vi "Sleep TC HL.vi"(8 "error in":errorcluster, 11 "Module ID":i32=-1) -> (0 "error out":errorcluster)   [LabVIEW 2020, in "NI DAQ.lvlib"]
doc: "Request to set the timeout of the TC HL to infinite.\n\n_____\nCreated using DQMH Framework: Event Scripter 7.1.1.1528."
uses:
  NI DAQ.lvlib
  Sleep TC HL Argument--cluster.ctl
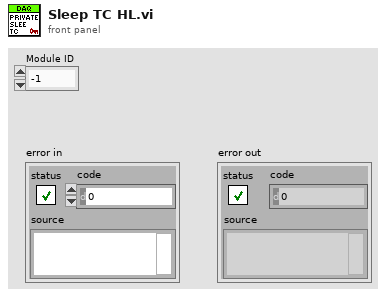
[diagram p1: front panel]
types:
  T1 = typedef "NI DAQ.lvlib/Sleep TC HL Argument--cluster.ctl" = cluster{"Module ID":i32, "Boolean":bool}
  T2 = typedef "NI DAQ.lvlib/Request Events--cluster.ctl" = cluster{"Stop Module":refnum<user-event>, "Show Panel":refnum<user-event>, "Hide Panel":refnum<user-event>, "Show Diagram":refnum<user-event>, "Get Module Execution Status":refnum<user-event>, "Set device name":refnum<user-event>, "Get channel list":refnum<user-event>, "Start task":refnum<user-event>, "Stop task":refnum<user-event>, "Write DO":refnum<user-event>, "Create DI channel":refnum<user-event>, "Read DI":refnum<user-event>, "Get task ref":refnum<user-event>, "Wake up HL":refnum<user-event>, "Sleep HL":refnum<user-event>, "Create AI channel":refnum<user-event>, "Read AI":refnum<user-event>, "Create AO channel":refnum<user-event>, "Write AO":refnum<user-event>, "Validate connection":refnum<user-event>, "Start continous acquisition":refnum<user-event>, "Stop continuous acquisition":refnum<user-event>, "Create DO channel":refnum<user-event>, "Create CI channel":refnum<user-event>, "Read CI":refnum<user-event>, "Get device model":refnum<user-event>, "Get device name":refnum<user-event>, "Create TC channel":refnum<user-event>, "Read TC":refnum<user-event>, "Start Continuous DI":refnum<user-event>, "Local Instance":T3, "Stop continuous DI":refnum<user-event>, "Private.Sleep DI HL":refnum<user-event>, "Start continuous AI":refnum<user-event>, "Private.Wake AI HL":refnum<user-event>, "Stop continuous AI":refnum<user-event>, "Private.Sleep AI HL":refnum<user-event>, "Start continuous TC":refnum<user-event>, "Private.Wake TC HL":refnum<user-event>, "Stop continuous TC":refnum<user-event>, "Private.Sleep TC HL":refnum<user-event>}
  T3 = typedef "NI DAQ.lvlib/Local Instance Request Events--cluster.ctl" = cluster{"Wake DI HL":refnum<user-event>}
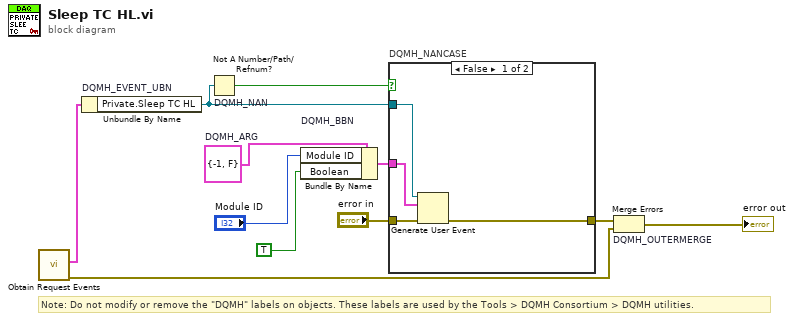
[diagram p0: block diagram]
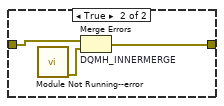
[diagram p2: hidden frame]
diagram:
  w5 = T1 {"Module ID"=-1, "Boolean"=FALSE}  # DQMH_ARG
  # "Note: Do not modify or remove the \"DQMH\" labels on objects. These labels are used by the Tools > DQMH Consortium > DQMH utilities."
  n1 = call "Obtain Request Events.vi"() -> ("error out"=w2:errorcluster, "NI DAQ Request Events"=w1:T2)  [unwired: 10 in]
  n2 = Unbundle By Name "DQMH_EVENT_UBN"(w1) -> ("Private.Sleep TC HL"=w7:refnum<user-event>)
  n3 = Not A Number/Path/Refnum? "DQMH_NAN"(number/path/refnum=w7) -> (NaN/Path/Refnum?=w8:bool)
  n4 = Bundle By Name "DQMH_BBN"(cluster=w5, "Module ID"="Module ID", "Boolean"=TRUE) -> (w9:T1)
  n5 = case "DQMH_NANCASE" shown="False" w8 {
    tunnel: "error in" -> [w15 w18]
    tunnel: [w14 w17] -> w6
    tunnel: w7 -> [w13 _]
    tunnel: w9 -> [w12 _]
    frame False {
      n6 = Generate User Event(user event=w13, event data cluster=w12, error in=w15) -> (error out=w14:errorcluster)  [unwired: 1 in, 1 out]
    }
    frame True {
      n7 = call "Module Not Running--error.vi"() -> ("error out"=w16:errorcluster)  [unwired: 11 in]
      n8 = Merge Errors "DQMH_INNERMERGE"(w18, w16) -> (w17:errorcluster)
    }
  }
  n9 = Merge Errors "DQMH_OUTERMERGE"(w6, w2) -> (→"error out":errorcluster)
